vi "Task Type.vi"(11 "DaqDigitalIn in":refnum<class "DaqDigitalIn.lvclass">) -> (2 "Task Type":string)   [LabVIEW 2020, in "VolatusDaq.lvlib" / "DaqDigitalIn.lvclass"]
uses:
  DaqDigitalIn.lvclass
  DaqDigitalIn.lvclass/DaqDigitalIn.ctl
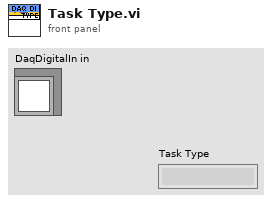
[diagram p1: front panel]
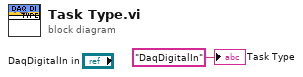
[diagram p0: block diagram]
diagram:
  "Task Type" <- "DaqDigitalIn" ("Task Type")
